vi "Teardown.vi"(11 "Hello World Event in":refnum<class "Hello World Event.lvclass">) -> (3 "Hello World Event out":refnum<class "Hello World Event.lvclass">)   [LabVIEW 2021, in "Hello World Event.lvlib" / "Hello World Event.lvclass"]
uses:
  Hello World Event.lvclass
  Hello World Event.lvclass/Hello World Event.ctl
  Actor/Event Actor/Event Actor.lvclass
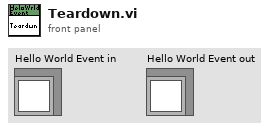
[diagram p1: front panel]
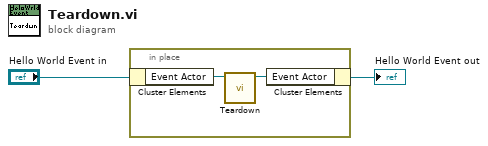
[diagram p0: block diagram]
diagram:
  n1 = in-place {
    n2 = in-place-cluster #1("Hello World Event in") -> ("Event Actor"=w4:refnum<class "Event Actor.lvclass">)
    n3 = call-dynamic "Teardown.vi"("Teardown in"=w4) -> ("Teardown out"=w3:refnum<class "Event Actor.lvclass">)  [unwired: 10 in]
    n4 = in-place-cluster #1("Event Actor"=w3) -> (→"Hello World Event out":refnum<class "Hello World Event.lvclass">)
  }
